vi "get_19052_IR_step_test_time.vi"(8 "error in (no error)":errorcluster, 10 "Step":u16=1 min=1 max=99 step=1, 11 "VISA resource in":refnum<visa-resource-name>) -> (0 "error out":errorcluster, 2 "IR total time":string, 3 "VISA resource out":refnum<visa-resource-name>)   [LabVIEW 2015]
doc: "This VI retrieves the test TIME of the selected step and mode."
uses:
  Type Definitions/get_19052_DC_IR_step_time_states.ctl
  Type Definitions/ac_dc_ir_control.ctl
  Type Definitions/dc_ir_control.ctl
panel:
  # "Get 19052 IR test time"
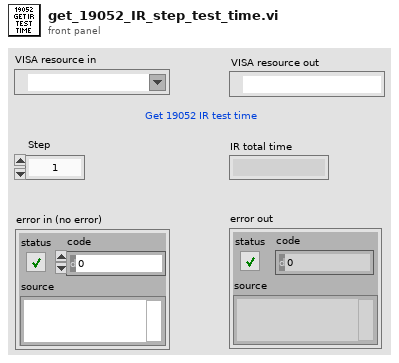
[diagram p1: front panel]
types:
  T1 = typedef "get_19052_DC_IR_step_time_states.ctl" = enum16{"Initilize", "get RAMP time", "get TIME", "get DWELL time", "get FALL time", "calc TOTAL time", "Error", "Shutdown"}
  T2 = cluster{"ramp time":dbl, "dwell time":dbl, "time":dbl, "fall time":dbl, "total time":string}
  T3 = typedef "ac_dc_ir_control.ctl" = enum16{"AC", "DC", "IR"}
  T4 = typedef "dc_ir_control.ctl" = enum16{"DC", "IR"}
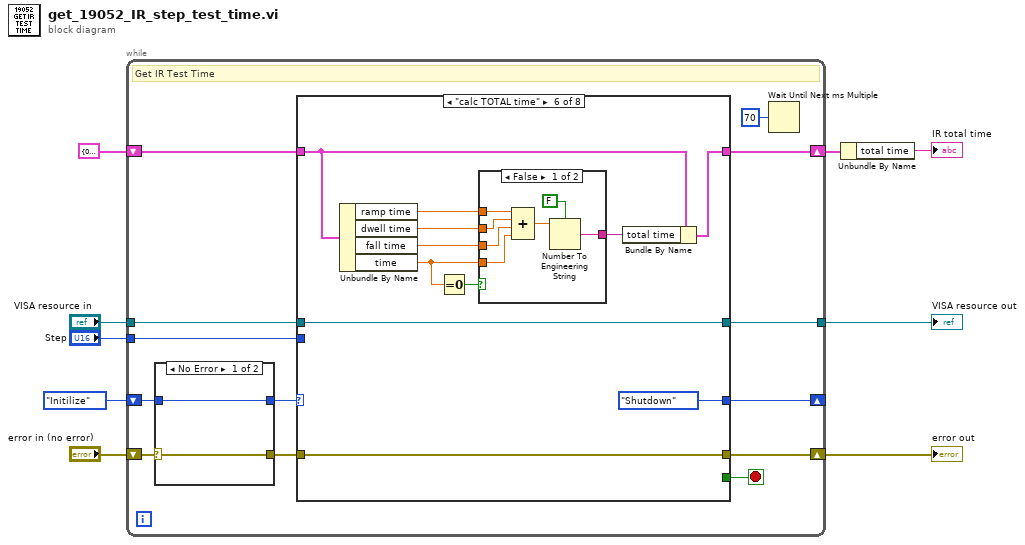
[diagram p0: block diagram]
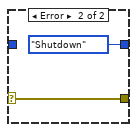
[diagram p2: hidden frame]
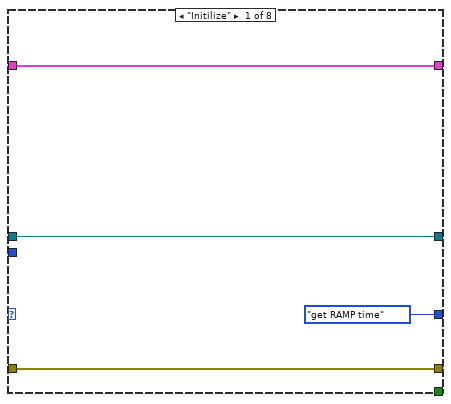
[diagram p3: hidden frame]
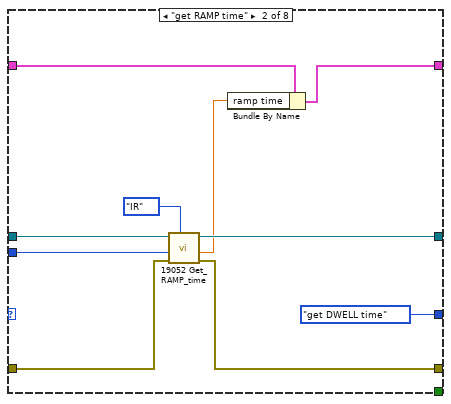
[diagram p4: hidden frame]
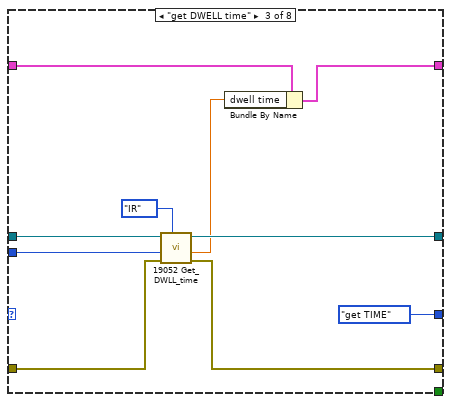
[diagram p5: hidden frame]
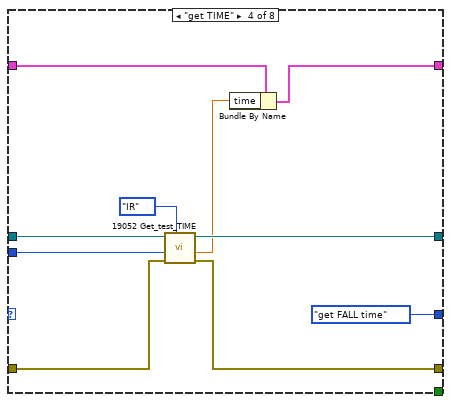
[diagram p6: hidden frame]
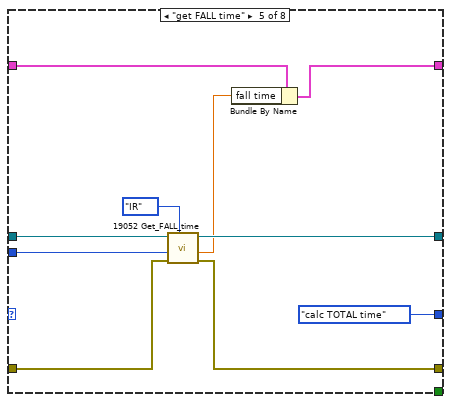
[diagram p7: hidden frame]
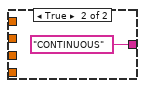
[diagram p8: hidden frame]
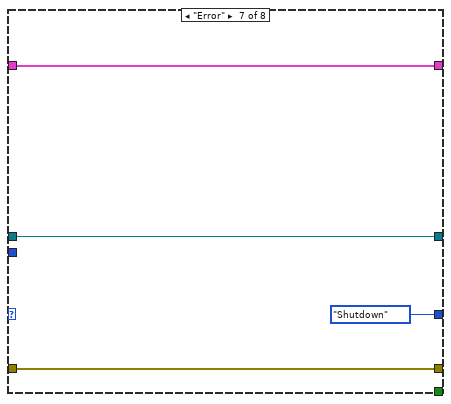
[diagram p9: hidden frame]
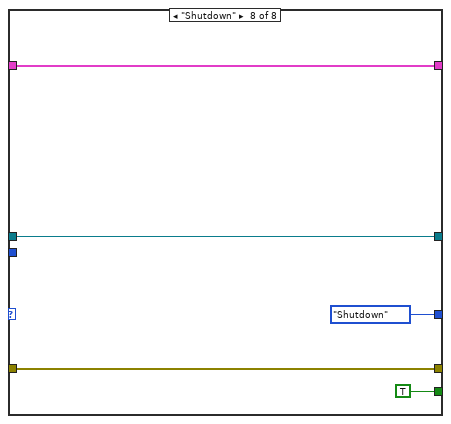
[diagram p10: hidden frame]
diagram:
  n1 = while {
    shift-right: [w22] -> _
    shift-left: get_19052_DC_IR_step_time_states."Initilize" ("States") -> [w13]
    tunnel: "VISA resource in" -> [w21]
    tunnel: [w20] -> w6
    shift-right: [w19] -> w8
    shift-left: "error in (no error)" -> [w16]
    shift-right: [w17] -> w3
    shift-left: T2 {"ramp time"=0.0, "dwell time"=0.0, "time"=0.0, "fall time"=0.0, "total time"=""} -> [w18]
    tunnel: "Step" -> [w12]
    stop <- w11 stop-if-true
    # "Get IR Test Time"
    n2 = case shown="No Error" w16 {
      selector: w16 -> [w24 w26]
      tunnel: [w24 w26] -> w15
      tunnel: [w23 get_19052_DC_IR_step_time_states."Shutdown" ("States")] -> w14
      tunnel: w13 -> [w23 _]
      frame No Error {
      }
      frame Error {
      }
    }
    n3 = case shown="\"calc TOTAL time\"" w14 {
      tunnel: [get_19052_DC_IR_step_time_states."get RAMP time" ("States") get_19052_DC_IR_step_time_states."get DWELL time" ("States") get_19052_DC_IR_step_time_states."get TIME" ("States") get_19052_DC_IR_step_time_states."get FALL time" ("States") get_19052_DC_IR_step_time_states."calc TOTAL time" ("States") get_19052_DC_IR_step_time_states."Shutdown" ("States") get_19052_DC_IR_step_time_states."Shutdown" ("States") get_19052_DC_IR_step_time_states."Shutdown" ("States")] -> w22
      tunnel: w21 -> [w30 w39 w50 w58 w68 w81 w93 w98]
      tunnel: [w30 w38 w49 w56 w66 w81 w93 w98] -> w20
      tunnel: w15 -> [w29 w37 w48 w57 w67 w80 w92 w97]
      tunnel: [w29 w36 w47 w55 w65 w80 w92 w97] -> w19
      tunnel: w18 -> [w28 w40 w45 w60 w70 w71 w91 w96]
      tunnel: [w28 w34 w44 w59 w69 w79 w91 w96] -> w17
      tunnel: w12 -> [_ w35 w41 w54 w64 _ _ _]
      tunnel: [_ _ _ _ _ _ _ TRUE] -> w11
      frame "Initilize" {
      }
      frame "get RAMP time" {
        n4 = call "19052 Get_RAMP_time.vi"("Mode"=ac_dc_ir_control."IR", "error in (no error)"=w37, "Step"=w35, "VISA resource in"=w39) -> ("error out"=w36:errorcluster, "RAMP time"=w33:dbl, "VISA resource out"=w38:refnum<visa-resource-name>)  [unwired: 5 in]
        n5 = Bundle By Name(cluster=w40, "ramp time"=w33) -> (w34:T2)
      }
      frame "get DWELL time" {
        n6 = call "19052 Get_DWLL_time.vi"("Mode"=dc_ir_control."IR", "error in (no error)"=w48, "Step"=w41, "VISA resource in"=w50) -> ("error out"=w47:errorcluster, "DWELL time"=w43:dbl, "VISA resource out"=w49:refnum<visa-resource-name>)  [unwired: 4 in, 1 out]
        n7 = Bundle By Name(cluster=w45, "dwell time"=w43) -> (w44:T2)
      }
      frame "get TIME" {
        n8 = call "19052 Get_test_TIME.vi"("Mode"=ac_dc_ir_control."IR", "error in (no error)"=w57, "Step"=w54, "VISA resource in"=w58) -> ("error out"=w55:errorcluster, "Test TIME"=w53:dbl, "VISA resource out"=w56:refnum<visa-resource-name>)  [unwired: 5 in]
        n9 = Bundle By Name(cluster=w60, "time"=w53) -> (w59:T2)
      }
      frame "get FALL time" {
        n10 = call "19052 Get_FALL_time.vi"("Mode"=ac_dc_ir_control."IR", "error in (no error)"=w67, "Step"=w64, "VISA resource in"=w68) -> ("error out"=w65:errorcluster, "FALL time"=w63:dbl, "VISA resource out"=w66:refnum<visa-resource-name>)  [unwired: 5 in]
        n11 = Bundle By Name(cluster=w70, "fall time"=w63) -> (w69:T2)
      }
      frame "calc TOTAL time" {
        n12 = Unbundle By Name(w71) -> ("ramp time"=w77:dbl, "dwell time"=w76:dbl, "fall time"=w75:dbl, "time"=w73:dbl)
        n13 = Equal To 0?(x=w73) -> (x = 0?=w74:bool)
        n14 = case shown="False" w74 {
          tunnel: w77 -> [w88 _]
          tunnel: w76 -> [w87 _]
          tunnel: w75 -> [w86 _]
          tunnel: [w83 "CONTINUOUS"] -> w72
          tunnel: w73 -> [w82 _]
          frame False {
            n15 = Compound Arithmetic op=ADD(w88, w87, w86, w82) -> (w85:dbl)
            n16 = Number To Engineering String(1:FALSE ("use system decimal point (T)"), 4:w85) -> (0:w83:string)  [unwired: 2 in]
          }
          frame True {
          }
        }
        n17 = Bundle By Name(cluster=w71, "total time"=w72) -> (w79:T2)
      }
      frame "Error" {
      }
      frame "Shutdown" {
      }
    }
    n18 = Wait Until Next ms Multiple(millisecond multiple=u32 70) -> ()  [unwired: 1 out]
  }
  "error out" <- w8
  "VISA resource out" <- w6
  n19 = Unbundle By Name(w3) -> ("total time"=→"IR total time":string)
